vi "Read Database.vi"(8 "error in (no error)":errorcluster, 10 "DB File Path":path, 11 "Database UI in":refnum<class "Database UI.lvclass">) -> (0 "error out":errorcluster, 3 "Database UI out":refnum<class "Database UI.lvclass">)   [LabVIEW 2023, in "Database UI.lvlib" / "Database UI.lvclass"]
uses:
  Database UI.lvclass
  Database UI.lvclass/Database UI.ctl
  <vilib>/drjdpowell/SQLite Library/SQL Statement/SQL Statement.lvclass/SQL Statement.ctl
  <vilib>/drjdpowell/SQLite Library/SQL Statement/Get Column Names.vi
  <vilib>/drjdpowell/SQLite Library/SQL Connection/Open (string).vi
  <vilib>/drjdpowell/SQLite Library/SQL Statement/Get Column Count.vi
  <vilib>/drjdpowell/SQLite Library/SQL Statement/Write Next Column.vi
  <vilib>/drjdpowell/SQLite Library/SQL Statement/Get Column Name.vi
  <vilib>/AdvancedString/Path To Command Line String.vi
  <vilib>/drjdpowell/SQLite Library/SQL Statement/Error Message.vi
  <vilib>/drjdpowell/SQLite Library/SQL Statement/Column String.vi
  <vilib>/drjdpowell/SQLite Library/SQL Connection/Connection.lvclass
  <vilib>/drjdpowell/SQLite Library/SQL Connection/Open (path).vi
  <vilib>/drjdpowell/SQLite Library/SQL Statement/SQL Statement.lvclass
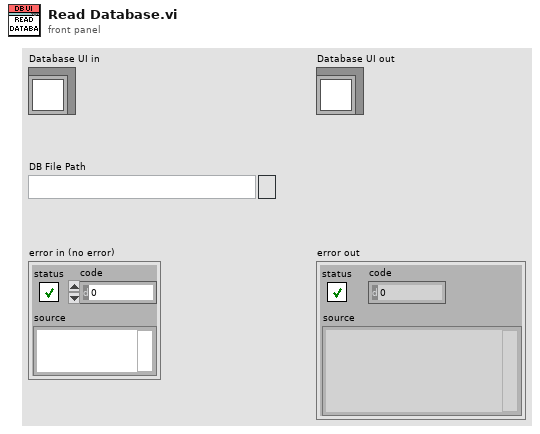
[diagram p1: front panel]
types:
  T1 = enum16{"New or existing", "Existing", "Read only"}
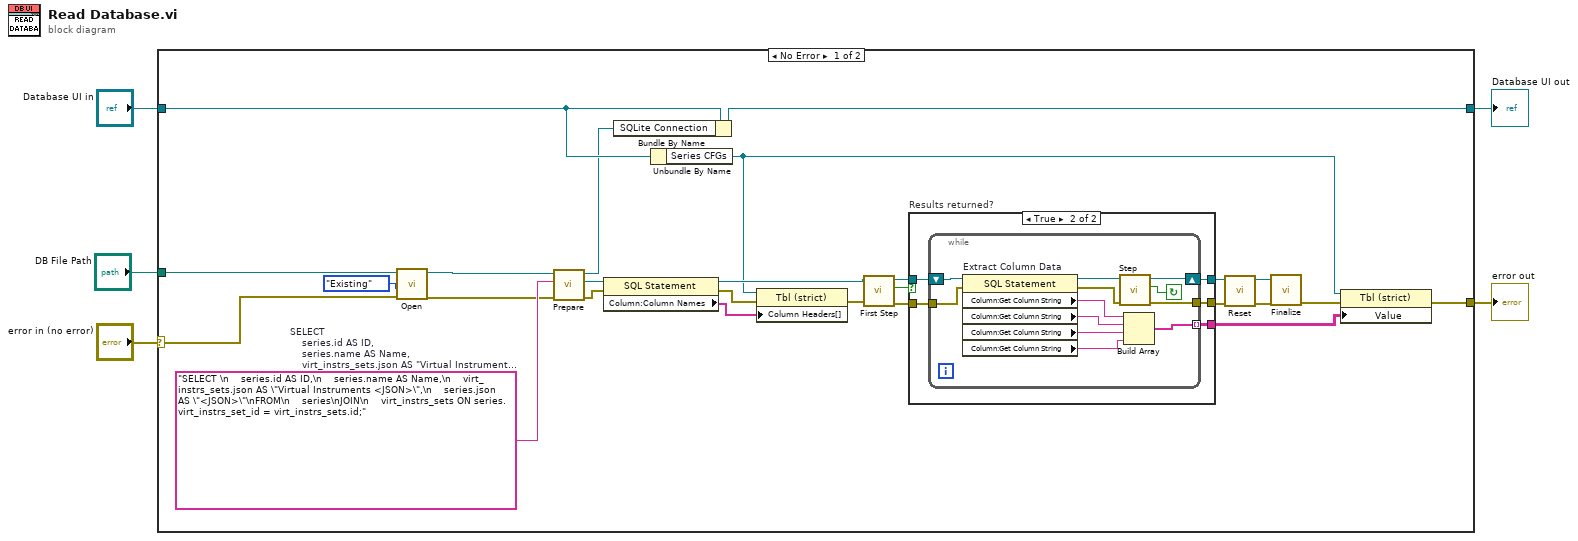
[diagram p0: block diagram]
diagram:
  n1 = case shown="No Error" "error in (no error)" {
    selector: "error in (no error)" -> [w31 w51]
    tunnel: [w30 w52] -> w3
    tunnel: "Database UI in" -> [w10 w52]
    tunnel: "DB File Path" -> [w7 _]
    tunnel: [w11 w51] -> w1
    frame No Error {
      w14 = "SELECT \n    series.id AS ID,\n    series.name AS Name,\n    virt_instrs_sets.json AS \"Virtual Instruments <JSON>\",\n    series.json AS \"<JSON>\"\nFROM\n    series\nJOIN\n    virt_instrs_sets ON series.virt_instrs_set_id = virt_instrs_sets.id;"  # SELECT      series.id AS ID,     series.name AS Name,     virt_instrs_sets.json AS "Virtual Instruments <JSON>",     series.json AS "<JSON>" FROM     series JOIN     virt_instrs_sets ON series.virt_instrs_set_id = virt_instrs_sets.id;
      n2 = call-poly <vilib>:"Open.vi"("error in (no error)"=w31, "File Option"=T1."Existing", "db file"=w7) -> ("error out"=w13:errorcluster, "SQLite Connection"=w12:refnum<class "Connection.lvclass">)  [unwired: 7 in]
      n3 = call <vilib>:"Prepare.vi"("error in (no error)"=w13, "SQL"=w14, "SQLite Connection in"=w12) -> ("error out"=w16:errorcluster, "SQL Statement"=w15:refnum<class "SQL Statement.lvclass">, "SQLite Connection"=w9:refnum<class "Connection.lvclass">)  [unwired: 4 in, 2 out]
      n4 = property class="SQL Statement"(reference=w15, error in=w16) -> (reference out=w20:refnum<class "SQL Statement.lvclass">, error out=w18:errorcluster, "Column:Column Names"=w17:string[])
      n5 = Bundle By Name(cluster=w10, "SQLite Connection"=w9) -> (w30:refnum<class "Database UI.lvclass">)
      n6 = Unbundle By Name(w10) -> ("Series CFGs"=w8:refnum<vi>)
      n7 = property on="Property Node" class="Tbl (strict)"(reference=w8, error in=w18, "Column Headers[]"=w17) -> (error out=w19:errorcluster)  [unwired: 1 out]
      n8 = call <vilib>:"First Step.vi"("error in (no error)"=w19, "SQL Statement in"=w20) -> ("error out"=w23:errorcluster, "Row returned"=w21:bool, "SQL Statement"=w22:refnum<class "SQL Statement.lvclass">)  [unwired: 7 in]
      n9 = case "Results returned?" shown="True" w21 {
        tunnel: w22 -> [w32 w38]
        tunnel: w23 -> [w33 w37]
        tunnel: [w33 w36] -> w24
        tunnel: [w32 w35] -> w25
        tunnel: [_ w34] -> w26
        frame False {
        }
        frame True {
          n10 = while {
            shift-right: [w47] -> w35
            shift-left: w38 -> [w50]
            tunnel: w37 -> [w48]
            tunnel: [w44] -> w36
            tunnel: [w40] -> w34 mode=indexing
            stop <- w45 continue-if-true
            n11 = property on="Extract Column Data" class="SQL Statement"(reference=w50, error in=w48) -> (reference out=w49:refnum<class "SQL Statement.lvclass">, error out=w46:errorcluster, "Column:Get Column String"=w43:string, "Column:Get Column String"=w42:string, "Column:Get Column String"=w41:string, "Column:Get Column String"=w39:string)
            n12 = call <vilib>:"Step.vi"("error in (no error)"=w46, "SQL Statement in"=w49) -> ("error out"=w44:errorcluster, "Row returned"=w45:bool, "SQL Statement"=w47:refnum<class "SQL Statement.lvclass">)  [unwired: 7 in]
            n13 = Build Array(w43, w42, w41, w39) -> (w40:string[])
          }
        }
      }
      n14 = call <vilib>:"Reset.vi"("error in (no error)"=w24, "SQL Statement in"=w25) -> ("error out"=w28:errorcluster, "SQL Statement"=w27:refnum<class "SQL Statement.lvclass">)  [unwired: 8 in]
      n15 = call <vilib>:"Finalize.vi"("error in (no error)"=w28, "SQL Statement in"=w27) -> ("error out"=w29:errorcluster)  [unwired: 9 in]
      n16 = property class="Tbl (strict)"(reference=w8, error in=w29, "Value"=w26) -> (error out=w11:errorcluster)  [unwired: 1 out]
    }
    frame Error {
    }
  }
  "error out" <- w1
  "Database UI out" <- w3
